vi "Parse Path Array indexes.vi"(9 "error in (no error)":errorcluster, 11 "Path with leading Array element":string) -> (1 "error out":errorcluster, 2 "Indexes (empty means use all)":i32[](array[numeric]), 3 "Rest or Path":string)   [LabVIEW 2017, in "JSONtext.lvlib"]
uses:
  JSONtext.lvlib
  JSON Value Type.ctl
  Parsing State.ctl
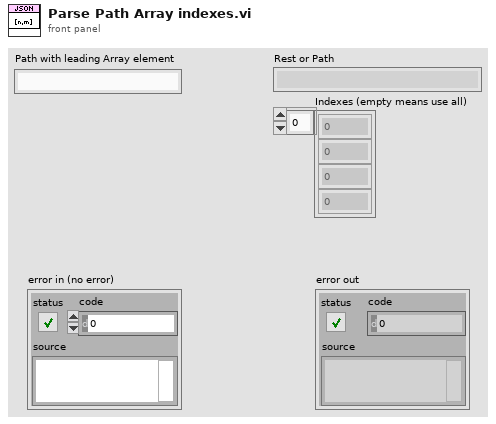
[diagram p1: front panel]
types:
  T1 = typedef "JSONtext.lvlib/Parsing State.ctl" = enum16{"Parser Error", "Object", "Array", "String", "Number/Other", "Leading Whitespace", "Object end", "Array end", "Value end"}
  T2 = typedef "JSONtext.lvlib/JSON Value Type.ctl" = enum16{"Not a JSON Value", "JSON Object", "JSON Array", "String", "Number", "true", "false", "null"}
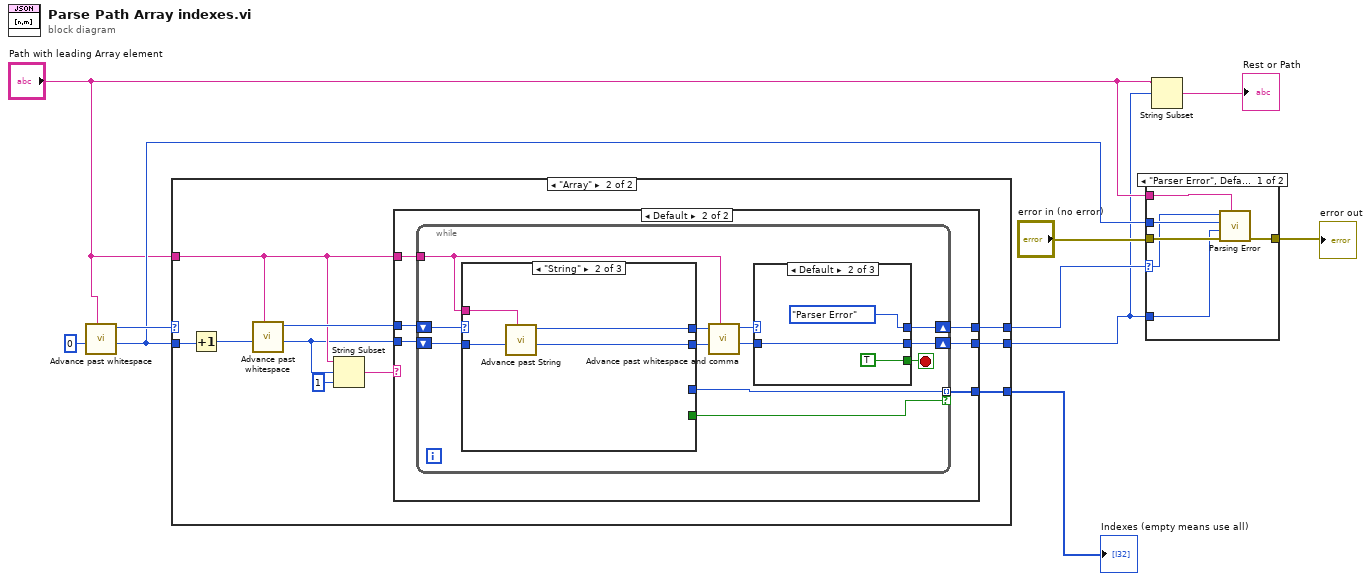
[diagram p0: block diagram]
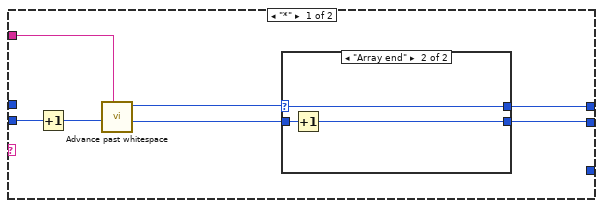
[diagram p4: hidden frame]
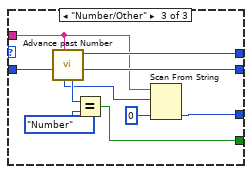
[diagram p7: hidden frame]
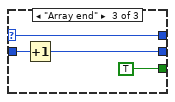
[diagram p9: hidden frame]
diagram:
  n1 = call "Advance past whitespace.vi"("JSON"="Path with leading Array element", "Offset"=0) -> ("Offset of first non-whitespace"=w6:i32, "Parser State"=w10:T1)  [unwired: 8 in]
  n2 = case shown="\"Array\"" w10 {
    selector: w10 -> [w11 _]
    tunnel: w6 -> [w12 w22]
    tunnel: "Path with leading Array element" -> [_ w19]
    tunnel: [_ w15] -> w5
    tunnel: [w12 w14] -> w2
    tunnel: [w11 w13] -> w7
    frame "Parser Error", Default {
    }
    frame "Array" {
      n3 = Increment(x=w22) -> (x+1=w20:i32)
      n4 = call "Advance past whitespace.vi"("JSON"=w19, "Offset"=w20) -> ("Offset of first non-whitespace"=w18:i32, "Parser State"=w21:T1)  [unwired: 8 in]
      n5 = String Subset(string=w19, offset (0)=w18, length (rest)=1 ("length (rest)")) -> (substring=w16:string)
      n6 = case shown="Default" w16 {
        tunnel: w21 -> [_ w40]
        tunnel: w19 -> [w23 w39]
        tunnel: w18 -> [w29 w38]
        tunnel: [_ w37] -> w15
        tunnel: [w25 w36] -> w14
        tunnel: [w24 w35] -> w13
        frame "*" {
          n7 = Increment(x=w29) -> (x+1=w28:i32)
          n8 = call "Advance past whitespace.vi"("JSON"=w23, "Offset"=w28) -> ("Offset of first non-whitespace"=w26:i32, "Parser State"=w27:T1)  [unwired: 8 in]
          n9 = case shown="\"Array end\"" w27 {
            selector: w27 -> [w31 w32]
            tunnel: w26 -> [w30 w34]
            tunnel: [w30 w33] -> w25
            tunnel: [w31 w32] -> w24
            frame "Parser Error", Default {
            }
            frame "Array end" {
              n10 = Increment(x=w34) -> (x+1=w33:i32)
            }
          }
        }
        frame Default {
          n11 = while {
            tunnel: w39 -> [w45]
            shift-right: [w50] -> w36
            shift-left: w38 -> [w43]
            shift-right: [w46] -> w35
            shift-left: w40 -> [w44]
            tunnel: [w42] -> w37 mode=indexing if=w41
            stop <- w49 stop-if-true
            n12 = case shown="\"String\"" w44 {
              selector: w44 -> [w54 _ _]
              tunnel: w43 -> [w53 w56 w66]
              tunnel: [w54 w58 w68] -> w48
              tunnel: [w53 w57 w67] -> w47
              tunnel: w45 -> [_ w55 w62]
              tunnel: [_ _ w59] -> w42
              tunnel: [_ _ w63] -> w41
              frame Default {
              }
              frame "String" {
                n13 = call "Advance past String.vi"("JSON"=w55, "Offset"=w56) -> ("Offset past match"=w57:i32, "State"=w58:T1)  [unwired: 7 in, 1 out]
              }
              frame "Number/Other" {
                n14 = call "Advance past Number.vi"("JSON"=w62, "Offset (0)"=w66) -> ("Offset past match"=w67:i32, "Parser State"=w68:T1, "JSON Value Type"=w65:T2, "Value start out"=w61:i32)  [unwired: 6 in]
                n15 = Equal?(x=w65, y=JSON_Value_Type."Number") -> (x = y?=w63:bool)
                n16 = Scan From String(input string=w62, initial scan location=w61, default 1=0) -> (output 1=w59:i32)  [unwired: 2 in, 3 out]
              }
            }
            n17 = call "Advance past whitespace and comma.vi"("JSON"=w45, "Offset"=w47, "State in"=w48) -> ("Offset past match"=w52:i32, "State"=w51:T1)  [unwired: 7 in]
            n18 = case shown="Default" w51 {
              selector: w51 -> [w69 _ w74]
              tunnel: [_ TRUE TRUE] -> w49
              tunnel: w52 -> [w70 w72 w76]
              tunnel: [w70 w72 w75] -> w50
              tunnel: [w69 Parsing_State."Parser Error" w74] -> w46
              frame "Number/Other" {
              }
              frame Default {
              }
              frame "Array end" {
                n19 = Increment(x=w76) -> (x+1=w75:i32)
              }
            }
          }
        }
      }
    }
  }
  "Indexes (empty means use all)" <- w5
  n20 = case shown="\"Parser Error\", Default" w7 {
    selector: w7 -> [w78 _]
    tunnel: "Path with leading Array element" -> [w83 _]
    tunnel: "error in (no error)" -> [w82 w84]
    tunnel: [w81 w84] -> w8
    tunnel: w6 -> [w80 _]
    tunnel: w2 -> [w79 _]
    frame "Parser Error", Default {
      n21 = call "Parsing Error.vi"("JSON"=w83, "error in (no error)"=w82, "Offset past match"=w79, "Value start"=w80, "State"=w78) -> ("error out"=w81:errorcluster)  [unwired: 6 in]
    }
    frame "Array end" {
    }
  }
  "error out" <- w8
  n22 = String Subset(string="Path with leading Array element", offset (0)=w2) -> (substring=→"Rest or Path":string)  [unwired: 1 in]
